vi "test Compare DFT Algorithms outputs 1.vi"(11 "Test Case In":refnum<class "test Compare DFT Algorithms outputs.lvclass">) -> (0 "error out":errorcluster, 3 "Test Case Out":refnum<class "test Compare DFT Algorithms outputs.lvclass">)   [LabVIEW 2023, in "test Compare DFT Algorithms outputs.lvclass"]
uses:
  test Compare DFT Algorithms outputs.lvclass
  C:/Program Files/National Instruments/LabVIEW 2023/vi.lib/Astemes/LUnit/Test Case.lvclass
  <vilib>/Astemes/LUnit/Test Case.lvclass/Test Case.ctl
  4993e8ee-a06a-463a-9684-69129f64d5ce.vi
  <vilib>/Astemes/LUnit/Append Pass Result.vi
  <vilib>/Astemes/LUnit/Append Fail Result.vi
  <vilib>/Astemes/LUnit/Describe Comparison.vi
  <vilib>/Astemes/LUnit/Compare Variants.vi
  <vilib>/Astemes/LUnit/Run In UI.vi
  <vilib>/Utility/error.llb/Clear Errors.vi
  <vilib>/Astemes/LUnit/Describe Variant.vi
  test Compare DFT Algorithms outputs.lvclass/test Compare DFT Algorithms outputs.ctl
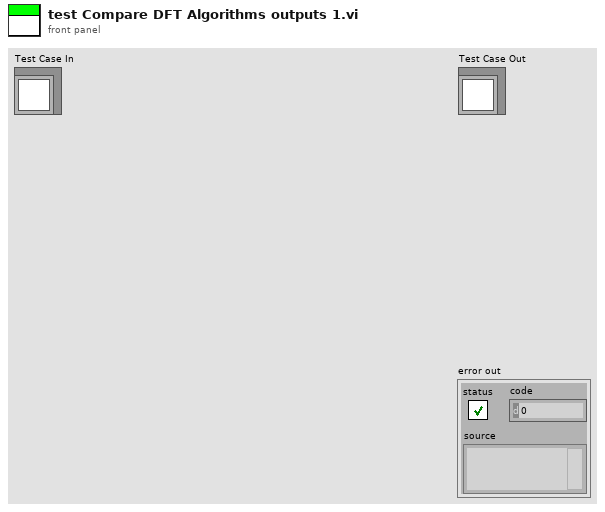
[diagram p1: front panel]
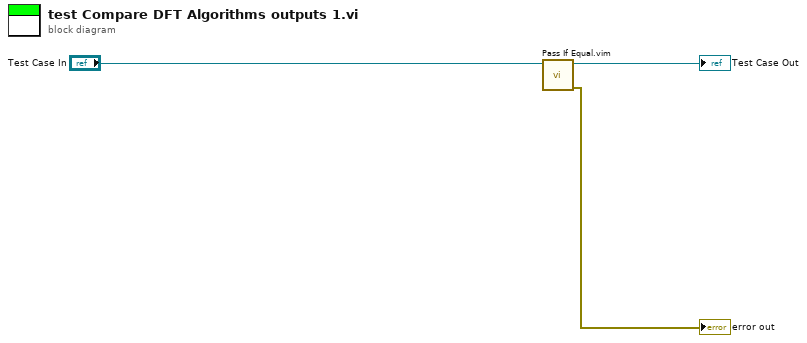
[diagram p0: block diagram]
diagram:
  n1 = call "Pass If Equal.vim"("LUnit Test Case In"="Test Case In") -> ("error out"=→"error out":errorcluster, "LUnit Test Case Out"=→"Test Case Out":refnum<class "test Compare DFT Algorithms outputs.lvclass">)  [unwired: 9 in]
